vi "Write Plot Legend.vi"(8 "error in (no error)":errorcluster, 10 "Plot Legend":bool=TRUE, 11 "2D Plot.lvclass in":refnum<class "2D Plot.lvclass">) -> (0 "error out":errorcluster, 3 "2D Plot.lvclass out":refnum<class "2D Plot.lvclass">)   [LabVIEW 2020, in "2D Plot.lvclass"]
uses:
  <vilib>/Math Plots/2D Math Plots/2D Plot/2D Plot/2D Plot.lvclass
  <vilib>/Math Plots/2D Math Plots/2D Plot/2D Plot/2D Plot.lvclass/2D Plot.ctl
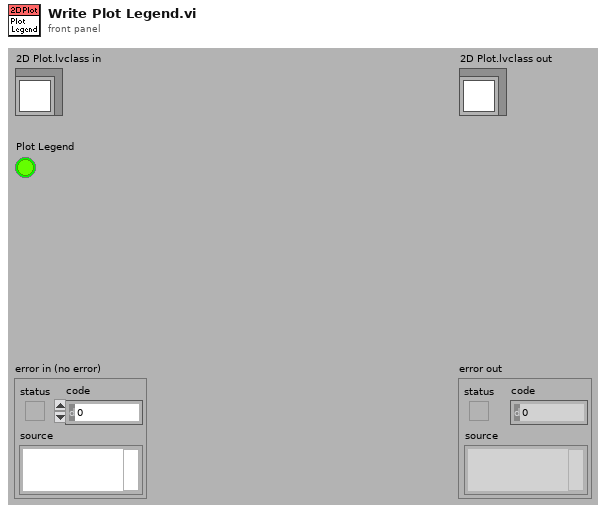
[diagram p1: front panel]
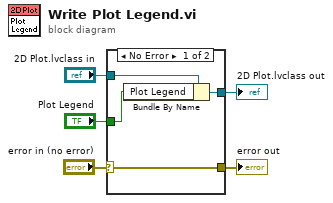
[diagram p0: block diagram]
diagram:
  n1 = case shown="No Error" "error in (no error)" {
    selector: "error in (no error)" -> [w9 w10]
    tunnel: [w9 w10] -> w4
    tunnel: [w7 w11] -> w2
    tunnel: "2D Plot.lvclass in" -> [w8 w11]
    tunnel: "Plot Legend" -> [w6 _]
    frame No Error {
      n2 = Bundle By Name(cluster=w8, "Plot Legend"=w6) -> (w7:refnum<class "2D Plot.lvclass">)
    }
    frame Error {
    }
  }
  "error out" <- w4
  "2D Plot.lvclass out" <- w2
